vi "rules update.vi"(0 "fuzzy system in":T1 {"user MF interpolating polynomials"."coa_x(y) coeff" format="%.4g"; "user MF interpolating polynomials"."Area(y) coeff" format="%.4g"; "user MF interpolating polynomials"."X(y) coeff" format="%.4g"; "user MF interpolating polynomials"."Y(x) coeff" format="%.4g"; "user MF interpolating polynomials"."Y" format="%.4g"; "user MF interpolating polynomials"."X" format="%.4g"; "defuzzification method" items=["Center of Area", "Modified Center of Area", "Center of Sums", "Center of Maximum", "Mean of Maximum"]; "rules"."consequents"."Var Index" min=0; "rules"."consequents"."Cond" items=["=", "!="]; "rules"."consequents"."MF Index" min=0; "rules"."antecedents"."Var Index" min=0; "rules"."antecedents"."Cond" items=["=", "!="]; "rules"."antecedents"."MF Index" min=0; "rules"."consequent implication" items=["Minimum", "Product"]; "rules"."antecedent connective" items=["AND (Minimum)", "AND (Product)", "OR (Maximum)", "OR (Probabilistic)"]; "output variables"."MFs"."shape" items=["Triangle", "Trapezoid", "Singleton", "Sigmoid", "Gaussian", "User-Defined"]; "input variables"."MFs"."shape" items=["Triangle", "Trapezoid", "Singleton", "Sigmoid", "Gaussian", "User-Defined"]}, 1 "Array in":i32[](array[numeric]), 2 "rule weights 2":dbl[](array[numeric]), 3 "rules as text":string[](array[string])) -> (16 "rules as text out":string[](array[string]))   [LabVIEW 2019]
uses:
  <vilib>/addons/Fuzzy Logic/TypeDefs/FL System.ctl
  <vilib>/addons/Fuzzy Logic/TypeDefs/FL Variable.ctl
  <vilib>/addons/Fuzzy Logic/TypeDefs/FL Membership Function.ctl
  <vilib>/addons/Fuzzy Logic/TypeDefs/FL Membership Function Shape.ctl
  <vilib>/addons/Fuzzy Logic/TypeDefs/FL Rule.ctl
  <vilib>/addons/Fuzzy Logic/TypeDefs/FL Antecedent.ctl
  <vilib>/addons/Fuzzy Logic/TypeDefs/FL Modifier.ctl
  <vilib>/addons/Fuzzy Logic/TypeDefs/FL Antecedent Connective.ctl
  <vilib>/addons/Fuzzy Logic/TypeDefs/FL Consequent.ctl
  <vilib>/addons/Fuzzy Logic/TypeDefs/FL Consequent Implication.ctl
  <vilib>/addons/Fuzzy Logic/TypeDefs/FL Defuzzification.ctl
  <vilib>/addons/Fuzzy Logic/TypeDefs/FL Interpolating polynomials.ctl
  <vilib>/addons/Fuzzy Logic/NI_Fuzzy_Logic_API.lvlib
panel:
  # "IF"
  # "THEN"
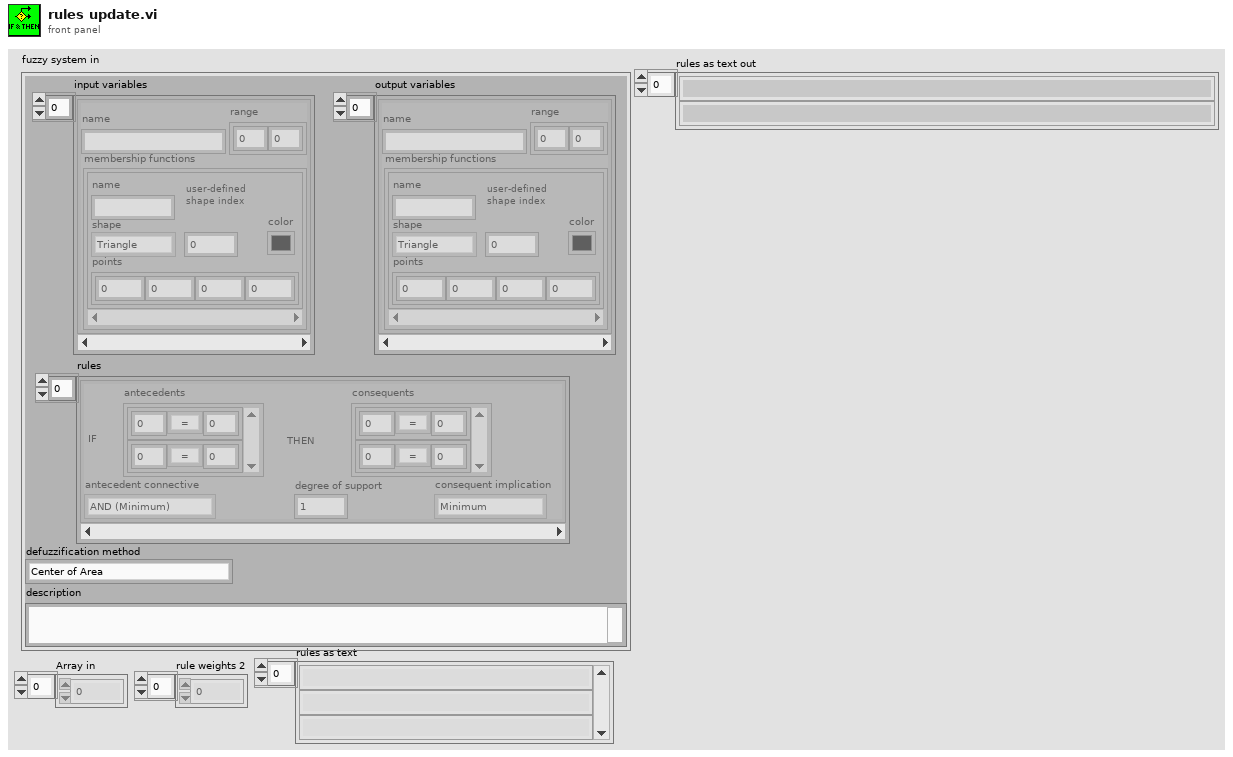
[diagram p1: front panel]
types:
  T1 = typedef "NI_Fuzzy_Logic_API.lvlib/FL System.ctl" = cluster{"input variables":T2[], "output variables":T2[], "rules":T5[], "defuzzification method":T11, "description":string, "user MF interpolating polynomials":T12[]}
  T2 = typedef "NI_Fuzzy_Logic_API.lvlib/FL Variable.ctl" = cluster{"name":string, "range":dbl[], "MFs":T3[]}
  T3 = typedef "NI_Fuzzy_Logic_API.lvlib/FL Membership Function.ctl" = cluster{"name":string, "shape":T4, "points":dbl[], "color":u32, "user-defined shape index":i32}
  T4 = typedef "NI_Fuzzy_Logic_API.lvlib/FL Membership Function Shape.ctl" = u16
  T5 = typedef "NI_Fuzzy_Logic_API.lvlib/FL Rule.ctl" = cluster{"antecedents":T6[], "antecedent connective":T8, "consequents":T9[], "consequent implication":T10, "degree of support":dbl}
  T6 = typedef "NI_Fuzzy_Logic_API.lvlib/FL Antecedent.ctl" = cluster{"Var Index":i32, "MF Index":i32, "Cond":T7}
  T7 = typedef "NI_Fuzzy_Logic_API.lvlib/FL Modifier.ctl" = u16
  T8 = typedef "NI_Fuzzy_Logic_API.lvlib/FL Antecedent Connective.ctl" = u16
  T9 = typedef "NI_Fuzzy_Logic_API.lvlib/FL Consequent.ctl" = cluster{"Var Index":i32, "MF Index":i32, "Cond":T7}
  T10 = typedef "NI_Fuzzy_Logic_API.lvlib/FL Consequent Implication.ctl" = u16
  T11 = typedef "NI_Fuzzy_Logic_API.lvlib/FL Defuzzification.ctl" = u16
  T12 = typedef "NI_Fuzzy_Logic_API.lvlib/FL Interpolating polynomials.ctl" = cluster{"X":dbl[], "Y":dbl[], "Y(x) coeff":dbl[][], "X(y) coeff":dbl[][], "Area(y) coeff":dbl[][], "coa_x(y) coeff":dbl[][]}
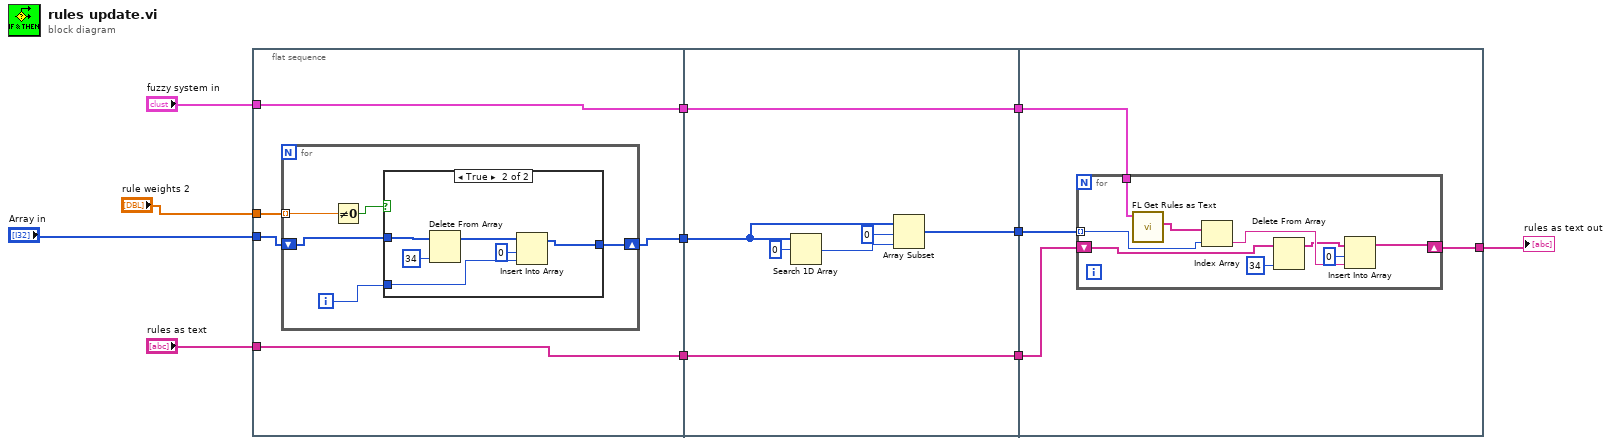
[diagram p0: block diagram]
diagram:
  n1 = flat-sequence {
    tunnel: "Array in" -> [w16]
    tunnel: "rule weights 2" -> [w15]
    tunnel: [w14] -> w9
    tunnel: [w13] -> w7
    tunnel: "fuzzy system in" -> [w13]
    tunnel: [w12] -> w4
    tunnel: "rules as text" -> [w12]
    tunnel: w9 -> [w32]
    tunnel: [w31] -> w8
    tunnel: w7 -> [w31]
    tunnel: [w30] -> w5
    tunnel: w4 -> [w30]
    tunnel: [w29] -> w2
    tunnel: w8 -> [w39]
    tunnel: w5 -> [w38]
    tunnel: w2 -> [w37]
    tunnel: [w36] -> w1
    frame #0 {
      n2 = for {
        tunnel: w15 -> [w21] mode=indexing
        shift-right: [w17] -> w14
        shift-left: w16 -> [w19]
        i -> [w18]
        n3 = Not Equal To 0?(x=w21) -> (x != 0?=w20:bool)
        n4 = case shown="True" w20 {
          tunnel: w19 -> [w22 w28]
          tunnel: w18 -> [_ w26]
          tunnel: [w22 w23] -> w17
          frame False {
          }
          frame True {
            n5 = Delete From Array(array=w28, index=34) -> (array with subset deleted=w25:i32[])  [unwired: 1 in, 1 out]
            n6 = Insert Into Array(array=w25, index=0, new element=w26) -> (w23:i32[])
          }
        }
      }
    }
    frame #1 {
      n7 = Search 1D Array(1D array=w32, element=i16 0) -> (index of element=w35:i32)  [unwired: 1 in]
      n8 = Array Subset(array=w32, index=0, length=w35) -> (w29:i32[])
    }
    frame #2 {
      n9 = for {
        tunnel: w37 -> [w40] mode=indexing
        tunnel: w39 -> [w48]
        shift-right: [w41] -> w36
        shift-left: w38 -> [w46]
        n10 = call <vilib>:"FL Get Rules as Text.vi"("fuzzy system in"=w48) -> ("rules as text"=w47:string[])  [unwired: 8 in, 2 out]
        n11 = Index Array(array=w47, index=w40) -> (element=w44:string)
        n12 = Delete From Array(array=w46, index=34) -> (array with subset deleted=w42:string[])  [unwired: 1 in, 1 out]
        n13 = Insert Into Array(array=w42, index=0, new element=w44) -> (w41:string[])
      }
    }
  }
  "rules as text out" <- w1
